vi "Synth Program.vi"(8 "Error In":errorcluster, 9 "Check if valid device":bool, 10 "Init":bool=TRUE, 11 "User configuration":T3={"DAQmx Device"="", "Variable amplitude frequency"=0.0, "Fixed amplitude frequency"=0.0, "Amplitude"=0.0, "Clock multiplier"=0, "Channel names (variable F)"=[], "Channel names (fixed F)"=[], "Group"="p", "Auto-update other modules"=FALSE, "Recorder module"="", "Lock-in module "=""} {"Amplitude" format="%#_6pV"; "Fixed amplitude frequency" format="%#_6pHz"; "Variable amplitude frequency" format="%#_6pHz"}) -> (0 "Error Out":errorcluster, 1 "Lockin parameters array":T1[](array[typedef]) {"DDS clock" format="%_17pHz"; "DDS modulus" format="0x%x (%d)"; "Phase" format="%#_gdeg"; "Frequency" format="%_17pHz"}, 2 "Actual ratios":T2 {"Clock" format="%_20p"; "F2" format="%_20p"; "F1" format="%_20p"; "Clock/F2" format="%_20g"; "Clock/F1" format="%_20g"}, 3 "Actual clock":ext format="%_20p", 4 "Checks out":bool)   [LabVIEW 2021]
uses:
  <resource>/objmgr/daqmx.rc
  Actual Settings.ctl
  NHMFL Synthesizer Configuration.ctl
  SoftwareLockin/Lockin Parameters.ctl
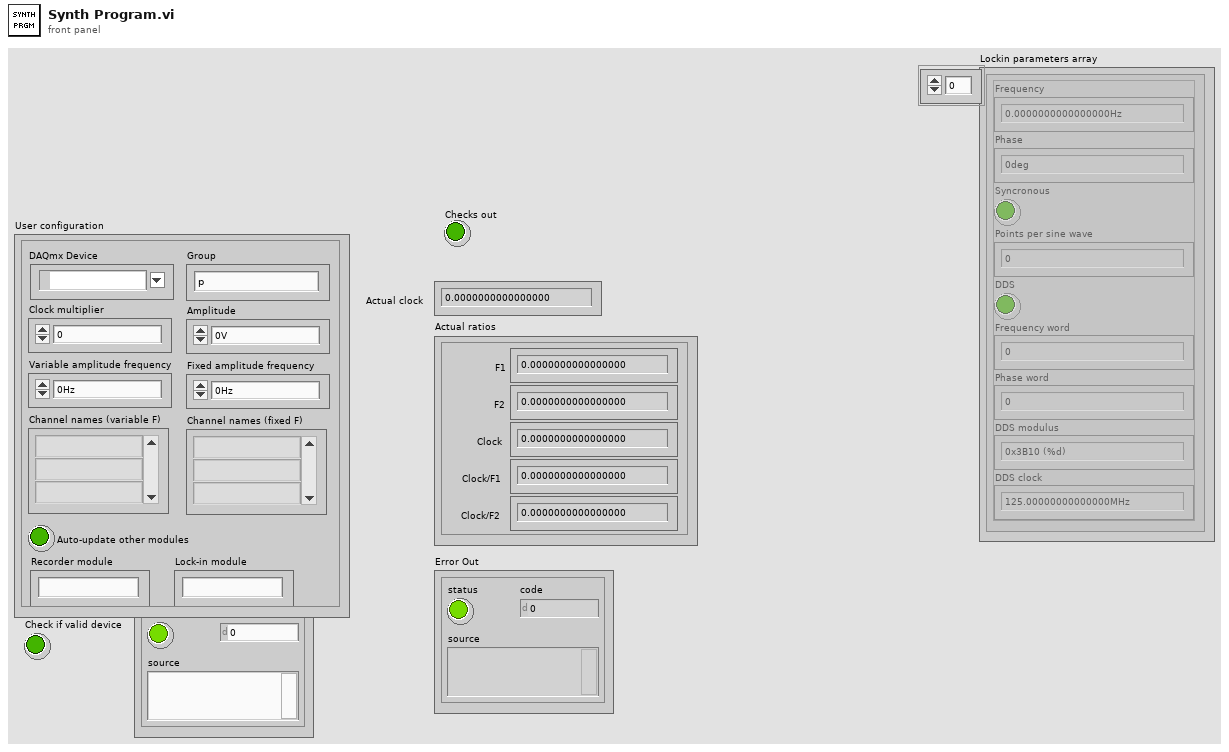
[diagram p1: front panel]
types:
  T1 = typedef "Lockin Parameters.ctl" = cluster{"Frequency":dbl, "Phase":dbl, "Syncronous":bool, "Points per sine wave":i32, "DDS":bool, "Frequency word":u32, "Phase word":u32, "DDS modulus":i64, "DDS clock":dbl}
  T2 = typedef "Actual settings.ctl" = cluster{"Clock/F1":ext, "Clock/F2":ext, "F1":ext, "F2":ext, "Clock":ext}
  T3 = typedef "NHMFL Synthesizer Configuration.ctl" = cluster{"DAQmx Device":tag, "Variable amplitude frequency":dbl, "Fixed amplitude frequency":dbl, "Amplitude":dbl, "Clock multiplier":i32, "Channel names (variable F)":string[], "Channel names (fixed F)":string[], "Group":string, "Auto-update other modules":bool, "Recorder module":string, "Lock-in module ":string}
  T4 = enum16{"Direct, clock*f1", "Direct, clock*f2", "Heterodyne"}
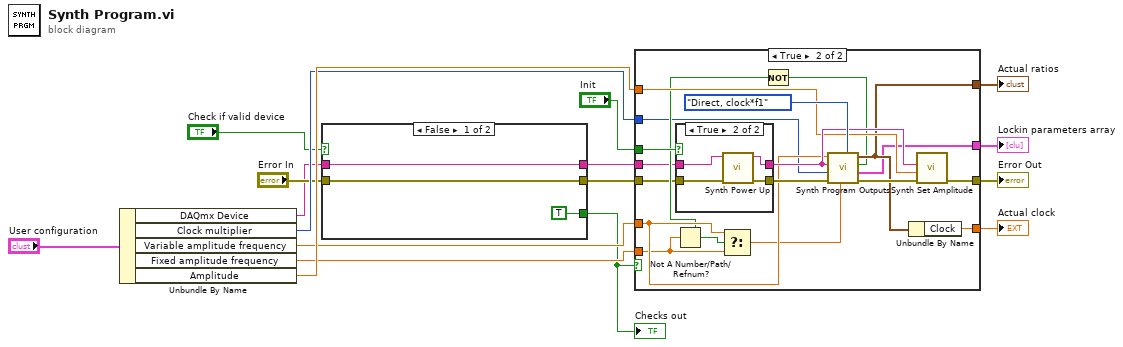
[diagram p0: block diagram]
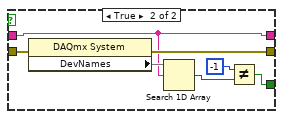
[diagram p4: hidden frame]
diagram:
  n1 = Unbundle By Name("User configuration") -> ("DAQmx Device"=w3:tag, "Clock multiplier"=w8:i32, "Variable amplitude frequency"=w10:dbl, "Fixed amplitude frequency"=w9:dbl, "Amplitude"=w14:dbl)
  n2 = case shown="False" "Check if valid device" {
    tunnel: w3 -> [w17 w20]
    tunnel: "Error In" -> [w18 w25]
    tunnel: [w18 w24] -> w5
    tunnel: [TRUE w21] -> w1
    tunnel: [w17 w20] -> w2
    frame False {
    }
    frame True {
      n3 = property class="DAQmx System"(error in=w25) -> (error out=w24:errorcluster, "DevNames"=w26)  [unwired: 1 in, 1 out]
      n4 = Search 1D Array(1D array=w26, element=w20) -> (index of element=w23:i32)  [unwired: 1 in]
      n5 = Not Equal?(x=-1, y=w23) -> (x != y?=w21:bool)
    }
  }
  "Checks out" <- w1
  n6 = case shown="True" w1 {
    tunnel: "Init" -> [_ w45]
    tunnel: w14 -> [_ w40]
    tunnel: [_ w39] -> w13
    tunnel: [_ w38] -> w12
    tunnel: [w27 w37] -> w11
    tunnel: w10 -> [_ w36]
    tunnel: w9 -> [_ w34]
    tunnel: w8 -> [_ w31]
    tunnel: [_ w30] -> w7
    tunnel: w5 -> [w27 w29]
    tunnel: w2 -> [_ w28]
    frame False {
    }
    frame True {
      n7 = Not A Number/Path/Refnum?(number/path/refnum=w34) -> (NaN/Path/Refnum?=w33:bool)
      n8 = case shown="True" w45 {
        tunnel: w28 -> [w47 w51]
        tunnel: w29 -> [w46 w50]
        tunnel: [w47 w49] -> w42
        tunnel: [w46 w48] -> w44
        frame False {
        }
        frame True {
          n9 = call "Synth Power Up.vi"("Error In"=w50, "DAQmx Device Name"=w51) -> ("Error Out"=w48:errorcluster, "DAQmx Device Name out"=w49:tag)  [unwired: 8 in]
        }
      }
      n10 = Select(t=w36, s=w33, f=w34) -> (s? t:f=w35:dbl)
      n11 = Not(x=w33) -> (.not. x?=w32:bool)
      n12 = call "Synth Program Outputs.vi"("Match clocks"=w32, "Mode"=T4."Direct, clock*f1", "IF (Hz)"=w35, "error in (no error)"=w44, "Clock Multiplier"=w31, "DAQmx Device Name"=w42, "f (Hz)"=w36) -> ("error out"=w41:errorcluster, "Lockin parameters array"=w30:T1[], "Actual ratios"=w39:T2)  [unwired: 2 in]
      n13 = Unbundle By Name(w39) -> ("Clock"=w38:ext)
      n14 = call "Synth Set Amplitude.vi"("error in (no error)"=w41, "0 to 2.1 VRMS"=w40, "DAQmx Device Name"=w42) -> ("error out"=w37:errorcluster)  [unwired: 8 in]
    }
  }
  "Actual ratios" <- w13
  "Error Out" <- w11
  "Actual clock" <- w12
  "Lockin parameters array" <- w7
